vi "Binary to ASCII - GPS Timestamp.vi"(0 "Binary File & Path":path, 3 "error in":errorcluster) -> (8 "data":dbl[][](array[numeric]), 10 "error out":errorcluster)   [LabVIEW 2013]
uses:
  <vilib>/Utility/file.llb/Write To Spreadsheet File (DBL).vi
  GPS Timekeeper Files/FPGA Timekeeper.lvlib
panel:
  out "LabVIEW time":timestamp
  out "Test File Path":path
  out "Waveform Graph":dbl[][](graph)
  out "size(s)":i32[](array[numeric])
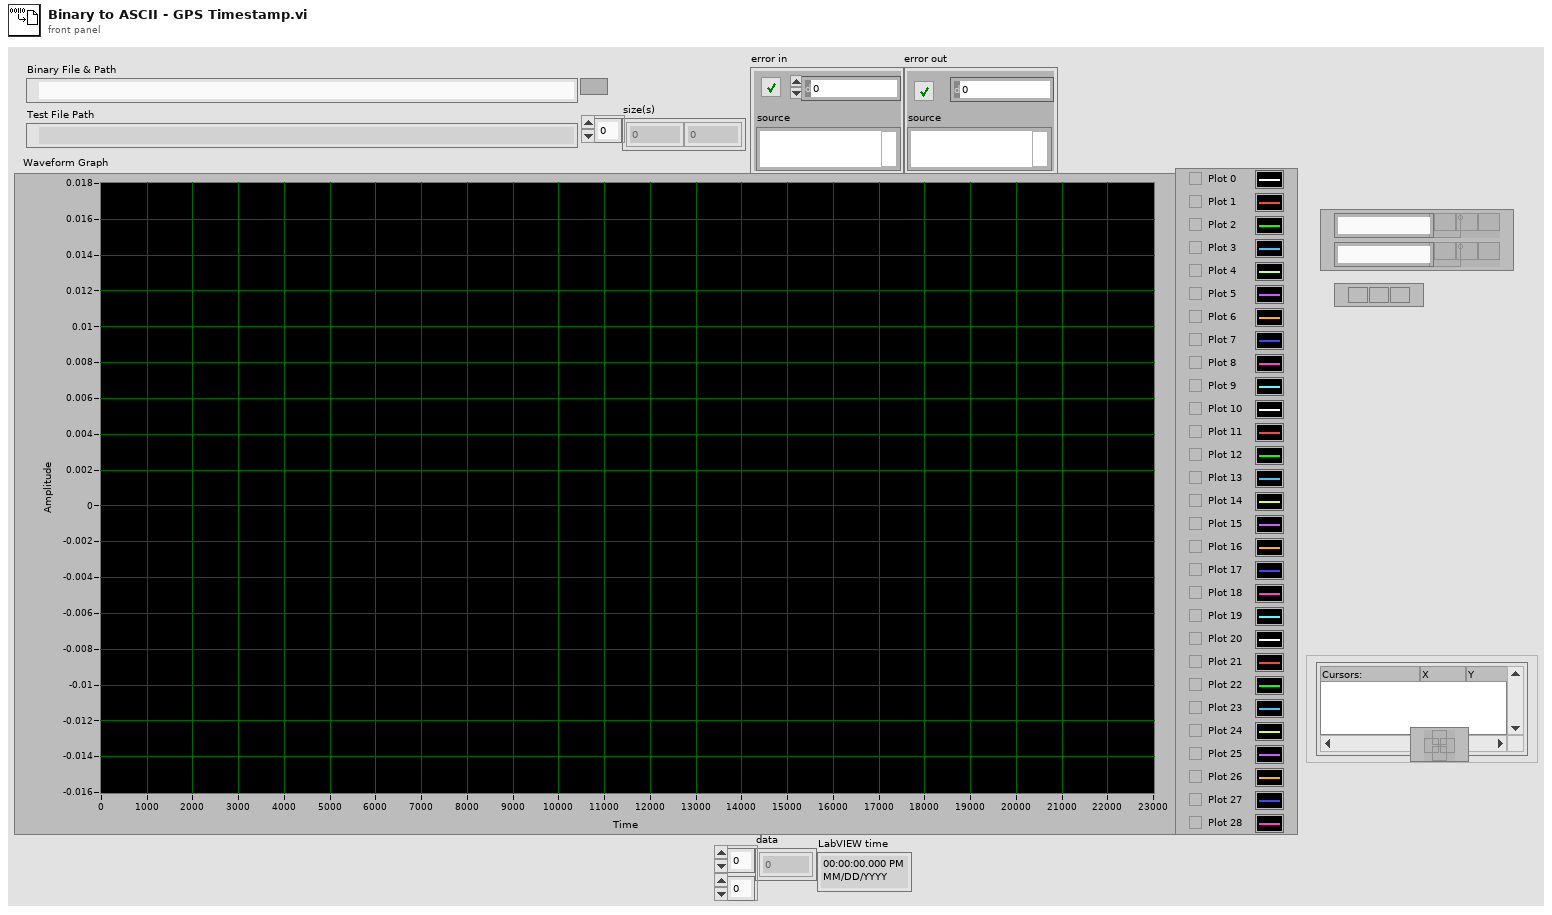
[diagram p1: front panel]
types:
  T1 = enum16{"open", "replace", "create", "open or create", "replace or create", "replace or create with confirmation"}
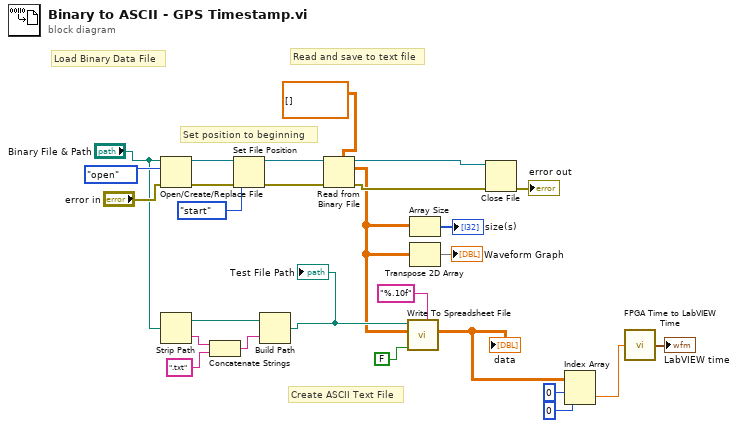
[diagram p0: block diagram]
diagram:
  # "Set position to beginning"
  # "Read and save to text file"
  # "Create ASCII Text File"
  # "Load Binary Data File"
  n1 = Open/Create/Replace File(file path (use dialog)="Binary File & Path", error in="error in", operation (0:open)=T1."open") -> (refnum out=w14:refnum<file>, error out=w16:errorcluster)  [unwired: 3 in, 1 out]
  n2 = Strip Path(path="Binary File & Path") -> (stripped path=w8:path, name=w10:string)
  n3 = Concatenate Strings(w10, ".txt" ("string")) -> (w7:string)
  n4 = Set File Position(refnum=w14, from (0:start)=enum16{"start", "end", "current"}."start", error in=w16) -> (refnum out=w13:refnum<file>, error out=w15:errorcluster)  [unwired: 1 in]
  n5 = Build Path(base path=w8, name or relative path=w7) -> (appended path=w6:path)
  "Test File Path" <- w6
  n6 = Read from Binary File(5:dbl[][] [], 8:w15, 11:w13) -> (0:w24:errorcluster, 2:w5:dbl[][], 3:w23:refnum<file>)  [unwired: 3 in, 1 out]
  "data" <- w5
  n7 = call-poly <vilib>:"Write To Spreadsheet File.vi"("format (%.3f)"="%.10f", "append to file? (new file:F)"=FALSE, "2D data"=w5, "file path (dialog if empty)"=w6) -> ()  [unwired: 4 in, 1 out]
  n8 = Array Size(array=w5) -> (size(s)=→"size(s)":i32[])
  n9 = Transpose 2D Array(2D array=w5) -> (transposed array=→"Waveform Graph":dbl[][])
  n10 = Close File(refnum=w23, error in=w24) -> (error out=→"error out":errorcluster)  [unwired: 1 out]
  n11 = Index Array(array=w5, index (row)=0, index (col)=0 ("disabled index (col)")) -> (element=w2:dbl)
  n12 = call "FPGA Time to LabVIEW Time.vi"("FPGA time (ns)"=w2) -> ("LabVIEW time"=→"LabVIEW time":timestamp)
